vi "Control - Industrial Control.vi"() -> ()   [LabVIEW 2013, in "Control Workspace Object.lvlib"]
doc: "Sample numeric display item."
uses:
  Control Workspace Object.lvlib
  <vilib>/NI Veristand/Display Template Support/Display Template Support.llb/cluster_Screen Item Settings.ctl
  <vilib>/NI Veristand/Display Template Support/Display Template Support.llb/cluster_Graph Scale Settings.ctl
  <vilib>/NI Veristand/Display Template Support/Display Template Support.llb/cluster_Graph Plot Settings.ctl
  NationalInstruments.VeriStand.SystemStorage
  <vilib>/NI Veristand/Display Template Support/Display Template Support.llb/enum_Display Template Handler Minimal To Widget Msg.ctl
  <vilib>/NI Veristand/Display Template Support/Display Template Support.llb/enum_Display Template Handler Minimal To Workspace.ctl
  Shared/Types/Workspace Object State Variables.ctl
  Types/UI.Refs.ctl
  Shared/Types/UDP Streaming Command Cluster.ctl
  Shared/Types/UDP Streaming State.ctl
  Shared/Types/Workspace Object Cached Settings.ctl
  <vilib>/NI Veristand/Execution/Workspace/WorkspaceAPI.ctl
  <vilib>/NI Veristand/Execution/Workspace/SystemStateRegEventRef.ctl
  <vilib>/NI Veristand/Execution/Workspace/SystemStateEventRef.ctl
  <vilib>/NI Veristand/Display Template Support/Display Template Support.llb/sub_Display Template Handler Custom.vi
  Shared/Constants.vi
  <vilib>/NI Veristand/Execution/Workspace/NI VeriStand - Get Multiple Channel Values.vi
  <vilib>/NI Veristand/Execution/Workspace/NI VeriStand - Set Single Channel Value.vi
  Shared/Control Addon Shared.lvlib
  <vilib>/NI Veristand/Execution/Workspace/NI_VS Workspace ExecutionAPI.lvlib
  NationalInstruments.VeriStand.ClientAPI
panel:
  in  "Manual Value":bool
  in  "Revert":bool
  in  "Apply":bool
  in  "Manual Output":dbl
  in  "Manual Control":bool
  in  "Setpoint":dbl
  in  "NIVS.System Definition Root":refnum<k24>
  in  "NIVS.Gateway IP Address":string
  in  "Hold":bool
  in  "Autoscale Y":bool=TRUE
  in  "Autoscale X":bool=TRUE
  out "Chart":waveform(dbl)[](graph)
  out "Control Name":string
  in  "Item.Data":T1
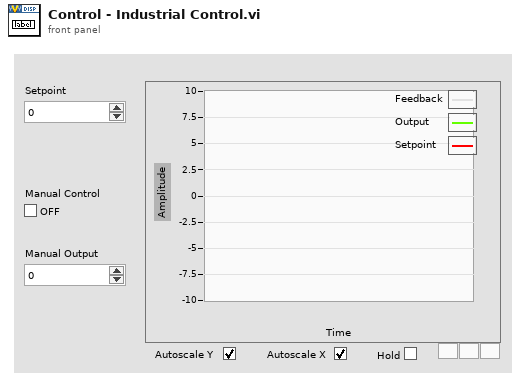
[diagram p1: front panel]
types:
  T1 = typedef "cluster_Screen Item Settings.ctl" = cluster{"Template VI":string, "Position X":i32, "Position Y":i32, "Custom":string, "Show Title Bar":bool, "ID":i32, "Always On Top":bool, "Allow Resize":bool, "Allow Minimize":bool, "Allow Close":bool, "Size to Screen":bool, "Screen.ID":i32, "State":enum16{"Normal", "New"}, "Title":string, "Window Bounds":cluster{"[0]":i16, "[1]":i16, "[2]":i16, "[3]":i16}, "Channel Ref":u64, "Unit":string, "Default Units?":bool, "Flash Limit?":bool, "Color 1":u32, "Color 2":u32, "Color 3":u32, "Color 4":u32, "Bck Color":u32, "Fore Color":u32, "Limit 1":dbl, "Limit 2":dbl, "Limit 3":dbl, "Limit 4":dbl, "Limit Mode 1":i32, "Limit Mode 2":i32, "Limit Mode 3":i32, "Limit Mode 4":i32, "Scale Precision":i32, "Scale Min":dbl, "Scale Max":dbl, "Format":i32, "Precision":i32, "Background Type":i32, "IDs":i32[], "Units":string[], "Labels":string[], "Scale Factor":dbl, "Scale Offset":dbl, "YScale Index":u32[], "XScale":T2, "YScales":T2[], "Plots":T3[], "Update Period":dbl, "History Length":dbl, "My.Ref":refnum<vi>, "Is Control?":bool, "Channel Paths":string[], "Custom Data":variant}
  T2 = typedef "cluster_Graph Scale Settings.ctl" = cluster{"Format":u8, "Precision":u8, "Fit":u8, "Label":string, "Use Default Label":bool, "Label Visible":bool, "Min":dbl, "Max":dbl}
  T3 = typedef "cluster_Graph Plot Settings.ctl" = cluster{"Bar Style":u8, "Fill To":i16, "Fill/PtColor":u32, "Line Style":u8, "Line Width":u8, "Color":u32, "Interp":u8, "Point Style":u8}
  T4 = typedef "Control Addon Shared.lvlib/Workspace Object State Variables.ctl" = cluster{"UI.Refs":T5, "Addon.GUID":string, "Addon.Name":string, "Addon.Type":enum16{"PID", "Industrial"}, "Data.UDPEngineQueue":refnum<queue>, "Data.Found?":bool, "Data.UDPChannels":string[], "Data.PreviousValues":dbl[], "Data.SlowChannels":string[], "Data.PendingChange?":bool, "CachedData.UserEvent":refnum<user-event>, "CachedData.Data":T6, "Workspace.Connected?":bool, "NIVS.SysDef":refnum<k24>, "NIVS.WorkspaceManager":T7, "NIVS.UserEventRefs":cluster{"Event Registration Refnum":refnum<event-registration>, "SystemChangeEventRef":T8}, "NIVS.SystemStateRefs":T9, "NIVS.LaunchRef":refnum<user-event>, "Setpoint Range":cluster{"Min":dbl, "Max":dbl}, "Output Range":cluster{"Min":dbl, "Max":dbl}}
  T5 = typedef "Control Addon Shared.lvlib/UI.Refs.ctl" = cluster{"Chart":refnum<vi>, "Manual Value":refnum<vi>, "Manual Output":refnum<vi>, "Revert":refnum<vi>, "Apply":refnum<vi>}
  T6 = typedef "Control Addon Shared.lvlib/Workspace Object Cached Settings.ctl" = cluster{"Path":string}
  T7 = typedef "NI_VS Workspace ExecutionAPI.lvlib/WorkspaceAPI.ctl" = refnum<k24>
  T8 = typedef "NI_VS Workspace ExecutionAPI.lvlib/SystemStateRegEventRef.ctl" = refnum<event-registration>
  T9 = typedef "NI_VS Workspace ExecutionAPI.lvlib/SystemStateEventRef.ctl" = cluster{"CustDatRef":refnum<user-event>, "EvtRef":refnum<k27>}
  T10 = typedef "enum_Display Template Handler Minimal To Workspace.ctl" = cluster{"Operation":enum16{"SetCustomData", "DeleteItem"}, "Data":variant}
  T11 = typedef "enum_Display Template Handler Minimal To Widget Msg.ctl" = enum16{"Stop", "LaunchConfigDialog"}
  T12 = typedef "Control Addon Shared.lvlib/UDP Streaming Command Cluster.ctl" = cluster{"Action":T13, "Channels":string[]}
  T13 = typedef "Control Addon Shared.lvlib/UDP Streaming State.ctl" = enum8{"Idle", "Start Acq", "Run", "Stop Acq", "Exit"}
  T14 = cluster{"Event Registration Refnum":refnum<event-registration>, "SystemChangeEventRef":T8}
  T15 = typedef "NI_VS Workspace ExecutionAPI.lvlib/SystemState.ctl" = u8
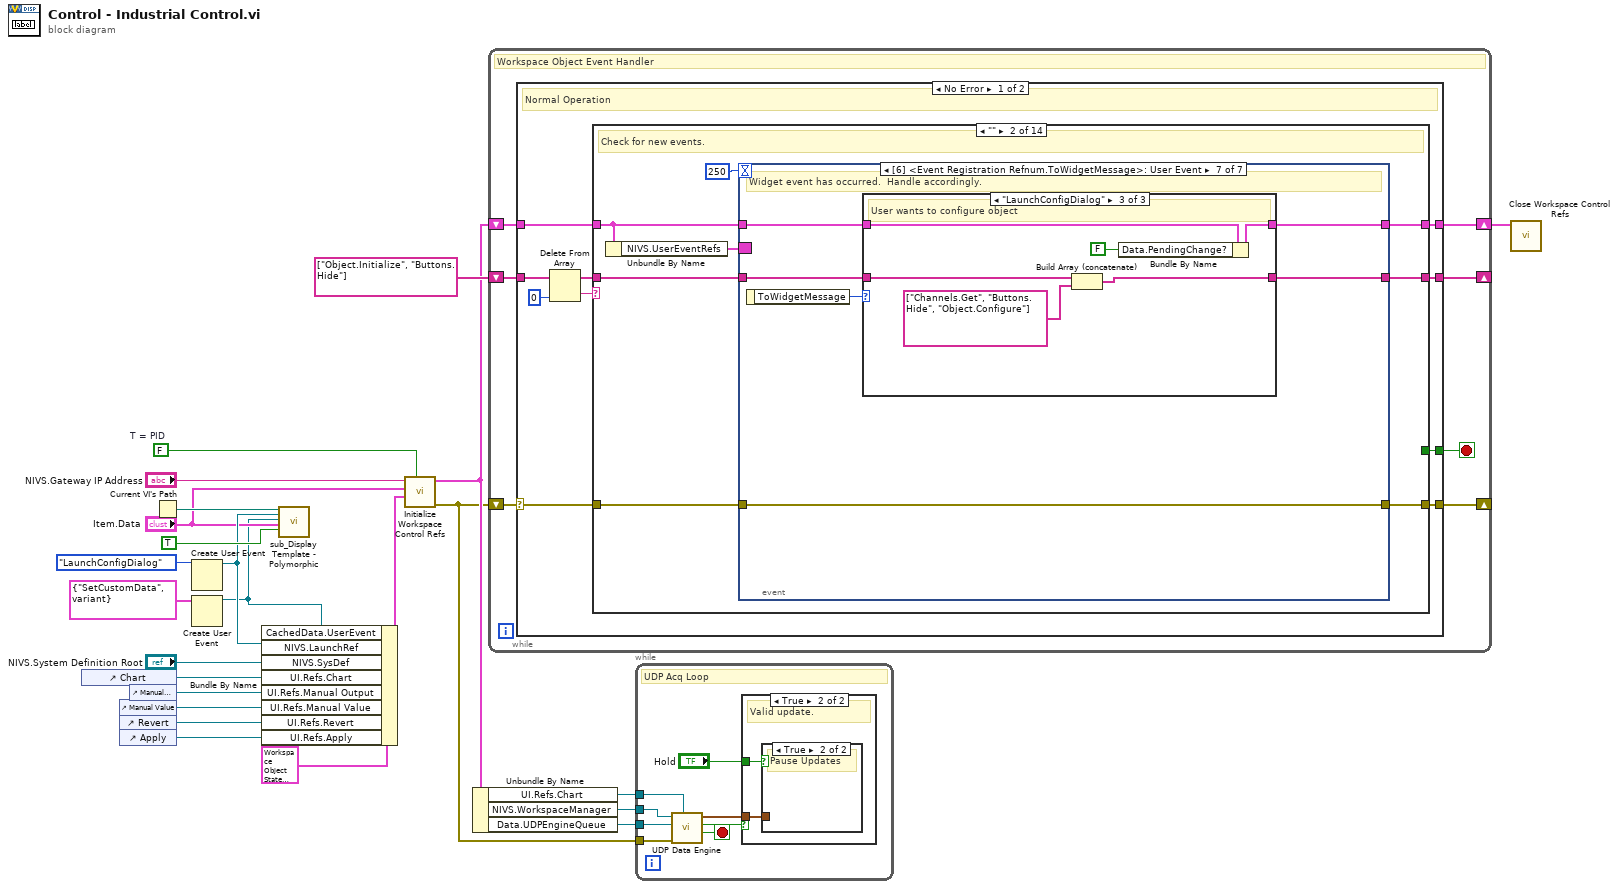
[diagram p0: block diagram]
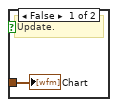
[diagram p3: hidden frame]
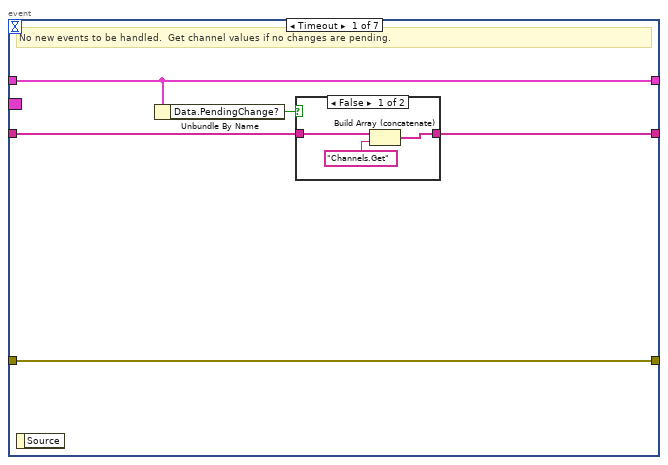
[diagram p5: hidden frame]
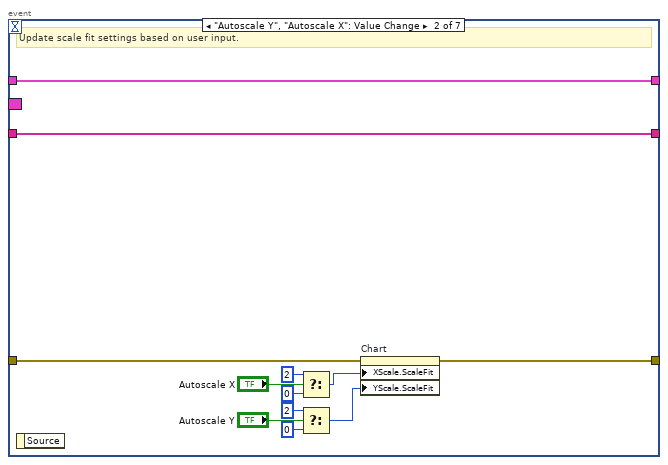
[diagram p7: hidden frame]
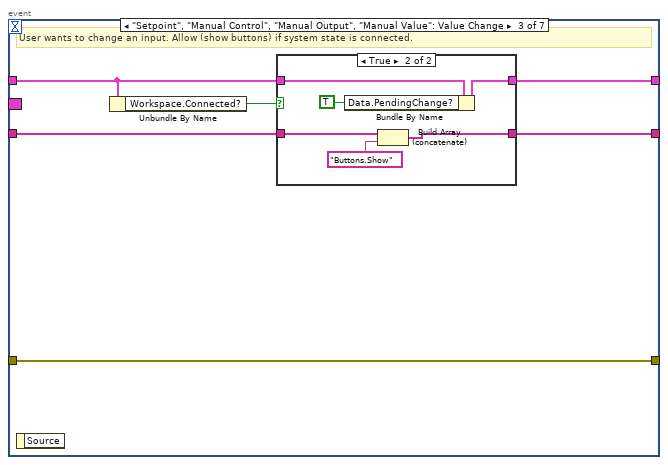
[diagram p8: hidden frame]
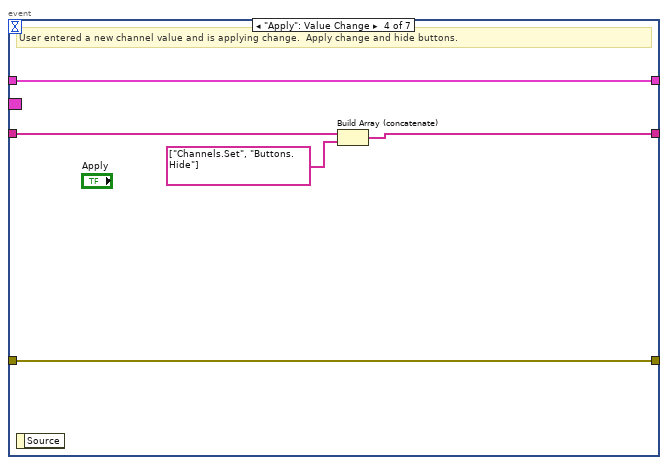
[diagram p10: hidden frame]
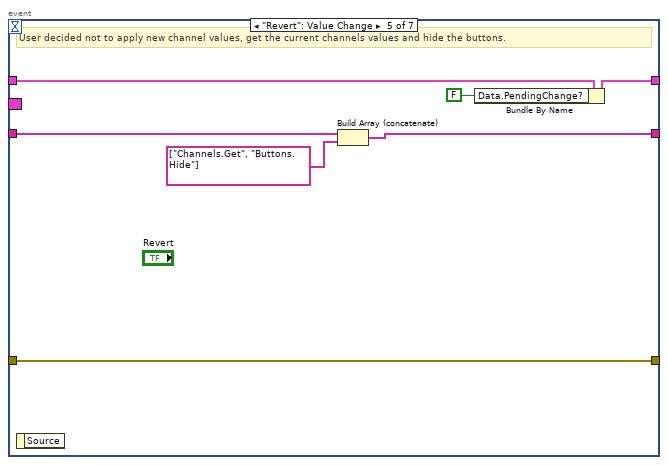
[diagram p11: hidden frame]
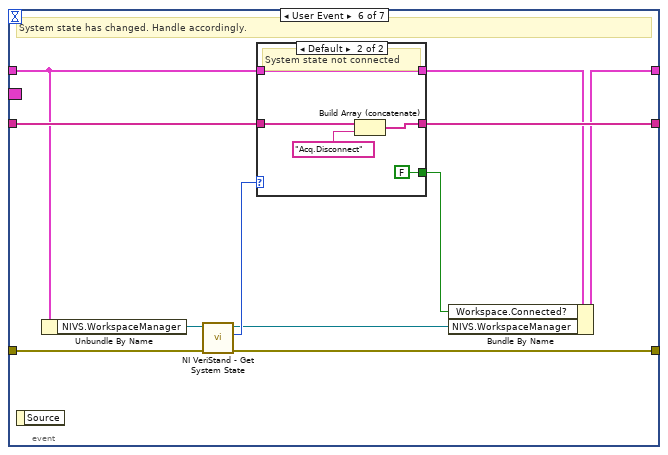
[diagram p12: hidden frame]
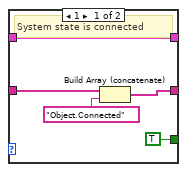
[diagram p13: hidden frame]
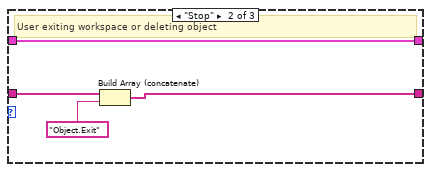
[diagram p15: hidden frame]
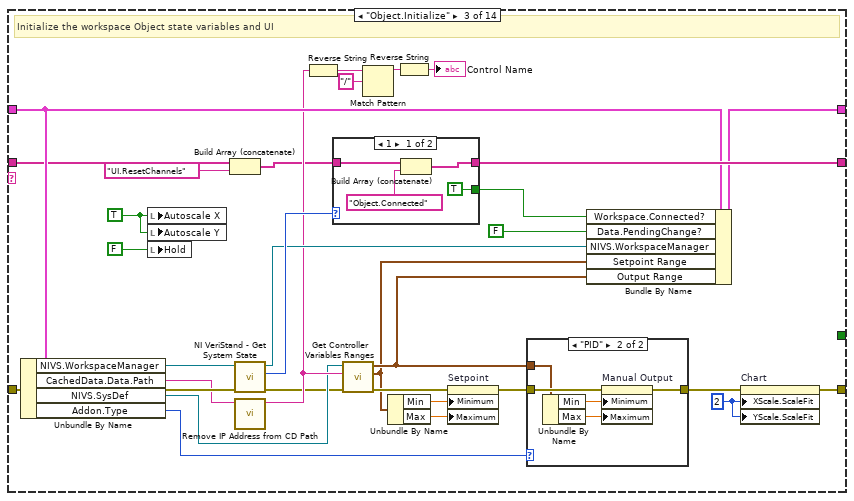
[diagram p16: hidden frame]
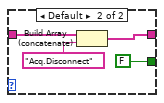
[diagram p18: hidden frame]
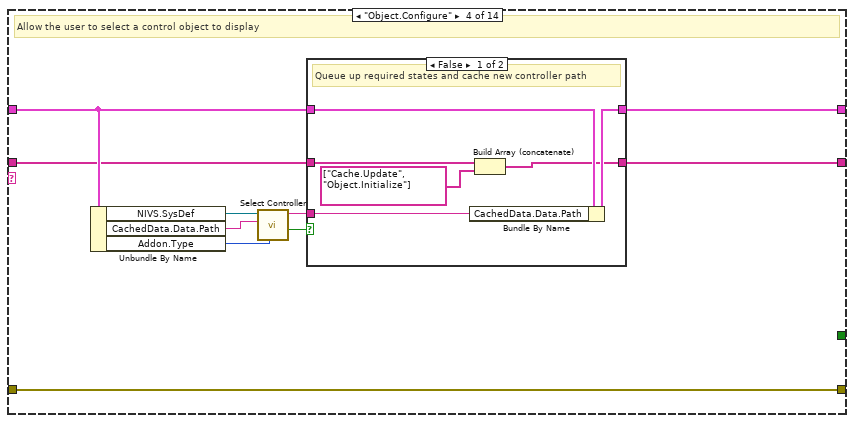
[diagram p19: hidden frame]
diagram:
  w6 = FALSE  # T = PID
  n1 = control-ref of="Chart"() -> (w12:refnum<vi>)
  n2 = control-ref of="Manual Value"() -> (w10:refnum<vi>)
  n3 = control-ref of="Revert"() -> (w9:refnum<vi>)
  n4 = control-ref of="Apply"() -> (w8:refnum<vi>)
  n5 = control-ref of="Manual Output"() -> (w11:refnum<vi>)
  n6 = Current VI's Path() -> (path=w22:path)
  n7 = Create User Event(user event datatype=enum_Display_Template_Handler_Minimal_To_Widget_Msg."LaunchConfigDialog" ("ToWidgetMessage")) -> (user event=w7:refnum<user-event>)  [unwired: 1 in, 1 out]
  n8 = Create User Event(user event datatype=T10 {"Operation"=enum."SetCustomData", "Data"=variant} ("Data")) -> (user event=w2:refnum<user-event>)  [unwired: 1 in, 1 out]
  n9 = Bundle By Name(cluster=T4 {"UI.Refs"={"Chart"=refnum, "Manual Value"=refnum, "Manual Output"=refnum, "Revert"=refnum, "Apply"=refnum}, "Addon.GUID"="", "Addon.Name"="", "Addon.Type"=enum."PID", "Data.UDPEngineQueue"=refnum, "Data.Found?"=FALSE, "Data.UDPChannels"=[], "Data.PreviousValues"=[], "Data.SlowChannels"=[], "Data.PendingChange?"=FALSE, "CachedData.UserEvent"=refnum, "CachedData.Data"={"Path"=""}, "Workspace.Connected?"=FALSE, "NIVS.SysDef"=refnum, "NIVS.WorkspaceManager"=refnum, "NIVS.UserEventRefs"={"Event Registration Refnum"=refnum, "SystemChangeEventRef"=refnum}, "NIVS.SystemStateRefs"={"CustDatRef"=refnum, "EvtRef"=refnum}, "NIVS.LaunchRef"=refnum, "Setpoint Range"={"Min"=0.0, "Max"=0.0}, "Output Range"={"Min"=0.0, "Max"=0.0}}, "CachedData.UserEvent"=w2, "NIVS.LaunchRef"=w7, "NIVS.SysDef"="NIVS.System Definition Root", "UI.Refs.Chart"=w12, "UI.Refs.Manual Output"=w11, "UI.Refs.Manual Value"=w10, "UI.Refs.Revert"=w9, "UI.Refs.Apply"=w8) -> (w4:T4)
  n10 = call-poly <vilib>:"sub_Display Template - Polymorphic.vi"("Parent.Path"=w22, "ToWidgetEvent"=w7, "ToWorkspace"=w2, "Item.Data"="Item.Data", "Resizable"=TRUE) -> ()  [unwired: 1 in, 14 out]
  n11 = call "Initialize Workspace Control Refs.vi"("T = PID"=w6, "State Variables in"=w4, "Item.Data"="Item.Data", "NIVS.Gateway IP Address"="NIVS.Gateway IP Address") -> ("error out"=w1:errorcluster, "State Variables out"=w15:T4)  [unwired: 6 in]
  n12 = Unbundle By Name(w15) -> ("UI.Refs.Chart"=w17:refnum<vi>, "NIVS.WorkspaceManager"=w16:T7, "Data.UDPEngineQueue"=w14:refnum<queue>)
  n13 = while {
    shift-right: [w29] -> _
    shift-left: string[] ["Object.Initialize", "Buttons.Hide"] -> [w30]
    shift-right: [w27] -> w19
    shift-left: w15 -> [w26]
    shift-right: [w28] -> _
    shift-left: w1 -> [w25]
    stop <- w31 stop-if-true
    # "Workspace Object Event Handler"
    n14 = case shown="No Error" w25 {
      selector: w25 -> [w32 w387]
      tunnel: [w41 _] -> w31
      tunnel: w30 -> [w39 w395]
      tunnel: [w36 w395] -> w29
      tunnel: [w35 w392] -> w28
      tunnel: [w34 w394] -> w27
      tunnel: w26 -> [w33 w394]
      frame No Error {
        # "Normal Operation"
        n15 = Delete From Array(array=w39, index=0) -> (deleted portion=w38:string, array with subset deleted=w37:string[])  [unwired: 1 in]
        n16 = case shown="\"\"" w38 {
          tunnel: [_ _ _ _ _ TRUE _ _ _ _ _ _ _ _] -> w41
          tunnel: [w44 w51 w168 w188 w212 w237 w244 w252 w254 w266 w272 w287 w347 w385] -> w36
          tunnel: w32 -> [w43 w49 w169 w194 w204 w232 w243 w247 w259 w262 w268 w284 w335 w384]
          tunnel: w37 -> [w44 w50 w140 w187 w223 w237 w244 w252 w260 w266 w272 w287 w347 w385]
          tunnel: w33 -> [w42 w45 w157 w192 w221 w229 w240 w251 w256 w265 w271 w277 w333 w382]
          tunnel: [w43 w48 w152 w194 w222 w231 w243 w246 w258 w261 w267 w283 w334 w384] -> w35
          tunnel: [w42 w47 w163 w191 w220 w229 w240 w251 w256 w265 w271 w282 w332 w382] -> w34
          frame Default {
            # "Do nothing."
          }
          frame "" {
            # "Check for new events."
            n17 = Unbundle By Name(w45) -> ("NIVS.UserEventRefs"=w46:T14)
            n18 = event shown="[6] <Event Registration Refnum.ToWidgetMessage>: User Event" {
              selector: w46 -> [_ _ _ _ _ _ _]
              dyn-events: _ -> [_ _ _ _ _ _ _]
              timeout: 250 -> [_ _ _ _ _ _ _]
              tunnel: [w55 w73 w76 w88 w96 w106 w125] -> w51
              tunnel: w50 -> [w56 w73 w77 w89 w97 w107 w124]
              tunnel: w49 -> [w57 w67 w79 w92 w99 w110 w123]
              tunnel: [w57 w66 w79 w92 w99 w109 w123] -> w48
              tunnel: [w54 w72 w78 w91 w94 w105 w121] -> w47
              tunnel: w45 -> [w54 w72 w75 w91 w95 w102 w122]
              event Timeout {
                # "No new events to be handled.  Get channel values if no changes are pending."
                n19 = event-data() -> ()  [unwired: 2 out]
                n20 = Unbundle By Name(w54) -> ("Data.PendingChange?"=w53:bool)
                n21 = case shown="False" w53 {
                  tunnel: w56 -> [w59 w61]
                  tunnel: [w58 w61] -> w55
                  frame False {
                    n22 = Build Array (concatenate)(w59, "Channels.Get") -> (w58:string[])
                  }
                  frame True {
                  }
                }
              }
              event "Autoscale Y", "Autoscale X": Value Change {
                # "Update scale fit settings based on user input."
                n23 = event-data() -> ()  [unwired: 2 out]
                n24 = Select(t=u8 2, s="Autoscale X", f=u8 0 ("X Scale.Scale Fit")) -> (s? t:f=w69:u8)
                n25 = Select(t=u8 2, s="Autoscale Y", f=u8 0 ("X Scale.Scale Fit")) -> (s? t:f=w62:u8)
                n26 = property on="Chart" class="WFChart (strict)"(error in=w67, "XScale.ScaleFit"=w69, "YScale.ScaleFit"=w62) -> (error out=w66:errorcluster)  [unwired: 1 in, 1 out]
              }
              event "Setpoint", "Manual Control", "Manual Output", "Manual Value": Value Change {
                # "User wants to change an input. Allow (show buttons) if system state is connected."
                n27 = event-data() -> ()  [unwired: 2 out]
                n28 = Unbundle By Name(w75) -> ("Workspace.Connected?"=w74:bool)
                n29 = case shown="True" w74 {
                  tunnel: w75 -> [w80 w86]
                  tunnel: [w80 w85] -> w78
                  tunnel: w77 -> [w81 w84]
                  tunnel: [w81 w82] -> w76
                  frame False {
                  }
                  frame True {
                    n30 = Bundle By Name(cluster=w86, "Data.PendingChange?"=TRUE ("Pending Change?")) -> (w85:T4)
                    n31 = Build Array (concatenate)(w84, "Buttons.Show") -> (w82:string[])
                  }
                }
              }
              event "Apply": Value Change {
                # "User entered a new channel value and is applying change.  Apply change and hide buttons."
                n32 = event-data() -> ()  [unwired: 2 out]
                n33 = Build Array (concatenate)(w89, string[] ["Channels.Set", "Buttons.Hide"]) -> (w88:string[])
              }
              event "Revert": Value Change {
                # "User decided not to apply new channel values, get the current channels values and hide the buttons."
                n34 = event-data() -> ()  [unwired: 2 out]
                n35 = Build Array (concatenate)(w97, string[] ["Channels.Get", "Buttons.Hide"]) -> (w96:string[])
                n36 = Bundle By Name(cluster=w95, "Data.PendingChange?"=FALSE ("Pending Change?")) -> (w94:T4)
              }
              event User Event {
                # "System state has changed. Handle accordingly."
                n37 = event-data() -> ()  [unwired: 2 out]
                n38 = Unbundle By Name(w102) -> ("NIVS.WorkspaceManager"=w101:T7)
                n39 = call <vilib>:"NI VeriStand - Get System State.vi"("error in (no error)"=w110, "WorkspaceManager in"=w101) -> ("error out"=w109:errorcluster, "System State"=w108:T15, "WorkspaceManager  out"=w100:T7)  [unwired: 5 in, 2 out]
                n40 = case shown="Default" w108 {
                  tunnel: w107 -> [w115 w120]
                  tunnel: [w114 w119] -> w106
                  tunnel: [w112 w117] -> w104
                  tunnel: w102 -> [w112 w117]
                  tunnel: [TRUE FALSE] -> w103
                  frame 1 {
                    # "System state is connected"
                    n41 = Build Array (concatenate)(w115, "Object.Connected") -> (w114:string[])
                  }
                  frame Default {
                    # "System state not connected"
                    n42 = Build Array (concatenate)(w120, "Acq.Disconnect") -> (w119:string[])
                  }
                }
                n43 = Bundle By Name(cluster=w104, "Workspace.Connected?"=w103, "NIVS.WorkspaceManager"=w100) -> (w105:T4)
              }
              event User Event {
                # "Widget event has occurred.  Handle accordingly."
                n44 = event-data() -> ("ToWidgetMessage"=w126:T11)  [unwired: 1 out]
                n45 = case shown="\"LaunchConfigDialog\"" w126 {
                  tunnel: [w128 w131 w137] -> w125
                  tunnel: w124 -> [w128 w132 w138]
                  tunnel: w122 -> [w127 w129 w134]
                  tunnel: [w127 w129 w133] -> w121
                  frame Default {
                    # "Do nothing."
                  }
                  frame "Stop" {
                    # "User exiting workspace or deleting object"
                    n46 = Build Array (concatenate)(w132, "Object.Exit") -> (w131:string[])
                  }
                  frame "LaunchConfigDialog" {
                    # "User wants to configure object"
                    n47 = Build Array (concatenate)(w138, string[] ["Channels.Get", "Buttons.Hide", "Object.Configure"]) -> (w137:string[])
                    n48 = Bundle By Name(cluster=w134, "Data.PendingChange?"=FALSE ("Pending Change?")) -> (w133:T4)
                  }
                }
              }
            }
          }
          frame "Object.Initialize" {
            w160 = u8 2 ("X Scale.Scale Fit")
            w161 = TRUE ("Autoscale X")
            # "Initialize the workspace Object state variables and UI"
            n49 = Unbundle By Name(w157) -> ("NIVS.WorkspaceManager"=w156:T7, "CachedData.Data.Path"=w150:string, "NIVS.SysDef"=w153:refnum<k24>, "Addon.Type"=w144:enum16{"PID", "Industrial"})
            n50 = local write "Autoscale X"(w161) -> ()
            n51 = local write "Autoscale Y"(w161) -> ()
            n52 = local write "Hold"(FALSE ("Hold")) -> ()
            n53 = Build Array (concatenate)(w140, "UI.ResetChannels") -> (w139:string[])
            n54 = call <vilib>:"NI VeriStand - Get System State.vi"("error in (no error)"=w169, "WorkspaceManager in"=w156) -> ("error out"=w151:errorcluster, "System State"=w170:T15, "WorkspaceManager  out"=w155:T7)  [unwired: 5 in, 2 out]
            n55 = call "Remove IP Address from CD Path.vi"("CD Path"=w150) -> ("Path"=w154:string)  [unwired: 10 in]
            n56 = Reverse String(1:w154) -> (0:w167:string)
            n57 = case shown="1" w170 {
              tunnel: w139 -> [w180 w184]
              tunnel: [w179 w183] -> w168
              tunnel: [TRUE FALSE] -> w162
              frame 1 {
                n58 = Build Array (concatenate)(w180, "Object.Connected") -> (w179:string[])
              }
              frame Default {
                n59 = Build Array (concatenate)(w184, "Acq.Disconnect") -> (w183:string[])
              }
            }
            n60 = call "Get Controller Variables Ranges.vi"("error in (no error)"=w151, "Path"=w154, "NIVS.SysDef Ref"=w153) -> ("error out"=w149:errorcluster, "Setpoint Range"=w142:cluster{"Min":dbl, "Max":dbl}, "Output Range"=w143:cluster{"Min":dbl, "Max":dbl})  [unwired: 6 in]
            n61 = Match Pattern(string=w167, regular expression="/") -> (before substring=w164:string)  [unwired: 1 in, 3 out]
            n62 = Unbundle By Name(w142) -> ("Min"=w148:dbl, "Max"=w147:dbl)
            n63 = Reverse String(1:w164) -> (0:→"Control Name":string)
            n64 = property on="Setpoint" class="DigNum (strict)"(error in=w149, "Minimum"=w148, "Maximum"=w147) -> (error out=w146:errorcluster)  [unwired: 1 in, 1 out]
            n65 = case shown="\"PID\"" w144 {
              tunnel: w146 -> [w171 w176]
              tunnel: [w171 w175] -> w145
              tunnel: w143 -> [_ w174]
              frame Default {
              }
              frame "PID" {
                n66 = Unbundle By Name(w174) -> ("Min"=w173:dbl, "Max"=w172:dbl)
                n67 = property on="Manual Output" class="DigNum (strict)"(error in=w176, "Minimum"=w173, "Maximum"=w172) -> (error out=w175:errorcluster)  [unwired: 1 in, 1 out]
              }
            }
            n68 = Bundle By Name(cluster=w157, "Workspace.Connected?"=w162, "Data.PendingChange?"=FALSE ("Pending Change?"), "NIVS.WorkspaceManager"=w155, "Setpoint Range"=w142, "Output Range"=w143) -> (w163:T4)
            n69 = property on="Chart" class="WFChart (strict)"(error in=w145, "XScale.ScaleFit"=w160, "YScale.ScaleFit"=w160) -> (error out=w152:errorcluster)  [unwired: 1 in, 1 out]
          }
          frame "Object.Configure" {
            # "Allow the user to select a control object to display"
            n70 = Unbundle By Name(w192) -> ("NIVS.SysDef"=w186:refnum<k24>, "CachedData.Data.Path"=w193:string, "Addon.Type"=w185:enum16{"PID", "Industrial"})
            n71 = call "Select Controller.vi"("Type"=w185, "CD Path"=w193, "NIVS.System Definition Root"=w186) -> ("Cancelled?"=w190:bool, "Custom Device Path Out"=w189:string)  [unwired: 6 in, 1 out]
            n72 = case shown="False" w190 {
              tunnel: w192 -> [w200 w201]
              tunnel: [w199 w201] -> w191
              tunnel: w189 -> [w198 _]
              tunnel: [w196 w202] -> w188
              tunnel: w187 -> [w197 w202]
              frame False {
                # "Queue up required states and cache new controller path"
                n73 = Bundle By Name(cluster=w200, "CachedData.Data.Path"=w198) -> (w199:T4)
                n74 = Build Array (concatenate)(w197, string[] ["Cache.Update", "Object.Initialize"]) -> (w196:string[])
              }
              frame True {
                # "User canceled"
              }
            }
          }
          frame "Object.Connected" {
            w209 = "/" ("string")
            # "System state is Connected. Get path to required channels and start UDP acquisition if channels found."
            n75 = Unbundle By Name(w221) -> ("NIVS.SysDef"=w205:refnum<k24>, "CachedData.Data.Path"=w219:string, "Addon.Name"=w206:string, "Addon.GUID"=w203:string)
            n76 = global read "Constants.vi" "Name.ManualControl"() -> (w218:string)
            n77 = global read "Constants.vi" "Name.Channels"() -> (w208:string)
            n78 = call "Remove IP Address from CD Path.vi"("CD Path"=w219) -> ("Path"=w217:string)  [unwired: 10 in]
            n79 = Concatenate Strings(w217, w209, w208, w209, w218) -> (w216:string)
            n80 = Concatenate Strings(w217, w209, w208, w209, w206) -> (w215:string)
            n81 = call "Get Dependent Nodes from SysDef Root.vi"("error in (no error)"=w204, "GUID"=w203, "Path"=w217, "SysDef Ref"=w205) -> ("error out"=w222:errorcluster, "Channels"=w211:string[], "Found"=w207:bool)  [unwired: 5 in]
            n82 = case shown="True" w207 {
              tunnel: w223 -> [w224 w227]
              tunnel: [w224 w226] -> w212
              frame False {
              }
              frame True {
                n83 = Build Array (concatenate)(w227, "Acq.Start") -> (w226:string[])
              }
            }
            n84 = Index Array(array=w211, index=2) -> (element=w213:string)
            n85 = Build Array(w213, w216, w215) -> (w210:string[])
            n86 = Bundle By Name(cluster=w221, "Data.Found?"=w207, "Data.UDPChannels"=w211, "Data.SlowChannels"=w210) -> (w220:T4)
          }
          frame "Object.Exit" {
            # "Stop current loop.  Queue Stop Acq and Exit to UDP loop."
            n87 = Unbundle By Name(w229) -> ("Data.UDPEngineQueue"=w228:refnum<queue>)
            n88 = Enqueue Element(queue=w228, element=T12 {"Action"=enum."Stop Acq", "Channels"=[]}, error in (no error)=w232) -> (queue out=w235:refnum<queue>, error out=w233:errorcluster)  [unwired: 1 in, 1 out]
            n89 = Enqueue Element(queue=w235, element=T12 {"Action"=enum."Exit", "Channels"=[]}, error in (no error)=w233) -> (error out=w231:errorcluster)  [unwired: 1 in, 2 out]
          }
          frame "Cache.Update" {
            # "Cache any data needing to be permenantly stored with the workspace object."
            n90 = Unbundle By Name(w240) -> ("CachedData.UserEvent"=w238:refnum<user-event>, "CachedData.Data"=w239:T6)
            n91 = Bundle By Name(cluster=T10 {"Operation"=enum."SetCustomData", "Data"=variant} ("event data"), "Data"=w239) -> (w241:T10)
            n92 = Generate User Event(user event=w238, event data cluster=w241) -> ()  [unwired: 2 in, 2 out]
          }
          frame "Acq.Start" {
            # "Send a Start Acq command to the UDP Loop.  Include the channels to  monitor."
            n93 = Unbundle By Name(w251) -> ("Data.UDPEngineQueue"=w245:refnum<queue>, "Data.UDPChannels"=w249:string[])
            n94 = Bundle By Name(cluster=T12 {"Action"=enum."Start Acq", "Channels"=[]}, "Channels"=w249) -> (w248:T12)
            n95 = Enqueue Element(queue=w245, element=w248, error in (no error)=w247) -> (error out=w246:errorcluster)  [unwired: 1 in, 2 out]
          }
          frame "Acq.Disconnect" {
            # "Send Stop Acq to the UDP Acq Loop.  Reset the UI."
            n96 = Unbundle By Name(w256) -> ("Data.UDPEngineQueue"=w255:refnum<queue>)
            n97 = Enqueue Element(queue=w255, element=T12 {"Action"=enum."Stop Acq", "Channels"=[]}, error in (no error)=w259) -> (error out=w258:errorcluster)  [unwired: 1 in, 2 out]
            n98 = Build Array (concatenate)(w260, "UI.ResetChannels") -> (w254:string[])
          }
          frame "Buttons.Hide" {
            w263 = FALSE ("Hold")
            # "Hide the apply and revert buttons from the user."
            n99 = property on="Apply" class="Bool"(error in=w262, "Visible"=w263) -> (error out=w264:errorcluster)  [unwired: 1 in, 1 out]
            n100 = property on="Revert" class="Bool"(error in=w264, "Visible"=w263) -> (error out=w261:errorcluster)  [unwired: 1 in, 1 out]
          }
          frame "Buttons.Show" {
            w269 = TRUE ("Hold")
            # "Show the apply and revert buttons to the user."
            n101 = property on="Apply" class="Bool"(error in=w268, "Visible"=w269) -> (error out=w270:errorcluster)  [unwired: 1 in, 1 out]
            n102 = property on="Revert" class="Bool"(error in=w270, "Visible"=w269) -> (error out=w267:errorcluster)  [unwired: 1 in, 1 out]
          }
          frame "Channels.Get" {
            # "Get the current slow speed channel values from VeriStand if no pending change, data paths are valid and system state is connected."
            n103 = Unbundle By Name(w277) -> ("Setpoint Range.Max"=w276:dbl, "Setpoint Range.Min"=w275:dbl, "Data.PendingChange?"=w278:bool, "Output Range.Max"=w274:dbl, "Output Range.Min"=w273:dbl, "Addon.Type"=w281:enum16{"PID", "Industrial"}, "Data.Found?"=w285:bool, "Workspace.Connected?"=w286:bool, "NIVS.WorkspaceManager"=w280:T7, "Data.SlowChannels"=w279:string[])
            n104 = case shown="False" w278 {
              tunnel: w286 -> [w309 _]
              tunnel: w285 -> [w303 _]
              tunnel: w284 -> [w300 w326]
              tunnel: [w299 w326] -> w283
              tunnel: [w298 w327] -> w282
              tunnel: w281 -> [w297 _]
              tunnel: w280 -> [w296 _]
              tunnel: w279 -> [w294 _]
              tunnel: w277 -> [w293 w327]
              tunnel: w276 -> [w291 _]
              tunnel: w275 -> [w290 _]
              tunnel: w274 -> [w289 _]
              tunnel: w273 -> [w288 _]
              frame False {
                # "No pending data change.  Allow for a get."
                n105 = Compound Arithmetic op=AND(w303, w309) -> (w304:bool)
                n106 = case shown="True" w304 {
                  tunnel: w300 -> [w319 w325]
                  tunnel: [w319 w324] -> w299
                  tunnel: w296 -> [w318 w323]
                  tunnel: [w318 w322] -> w295
                  tunnel: w294 -> [_ w321]
                  tunnel: [dbl[] [0.0, 0.0, 0.0] ("Values") w320] -> w308
                  frame False {
                    # "Do Nothing."
                  }
                  frame True {
                    # "Connected & paths valid"
                    n107 = call-poly <vilib>:"NI VeriStand - Get Channel Value.vi"("error in (no error)"=w325, "Channels"=w321, "WorkspaceManager in"=w323) -> ("error out"=w324:errorcluster, "Values"=w320:dbl[], "WorkspaceManager out"=w322:T7)  [unwired: 6 in]
                  }
                }
                n108 = Index Array(array=w308) -> (element #1=w307:dbl, element #2=w302:dbl, element #3=w301:dbl)  [unwired: 3 in]
                n109 = case shown="\"PID\"" w297 {
                  tunnel: w301 -> [w311 w316]
                  tunnel: w289 -> [_ w314]
                  tunnel: w288 -> [_ w313]
                  frame "Industrial" {
                    n110 = To Long Integer(number=w311) -> (32bit integer=w312:i32)
                    n111 = Not Equal To 0?(x=w312) -> (x != 0?=w310:bool)
                    n112 = local write "Manual Value"(w310) -> ()
                  }
                  frame "PID" {
                    n113 = In Range and Coerce(upper limit=w314, x=w316, lower limit=w313) -> (coerced(x)=w315:dbl)  [unwired: 1 out]
                    n114 = local write "Manual Output"(w315) -> ()
                  }
                }
                n115 = To Long Integer(number=w302) -> (32bit integer=w306:i32)
                n116 = In Range and Coerce(upper limit=w291, x=w307, lower limit=w290) -> (coerced(x)=w292:dbl)  [unwired: 1 out]
                n117 = Not Equal To 0?(x=w306) -> (x != 0?=w305:bool)
                n118 = local write "Setpoint"(w292) -> ()
                n119 = local write "Manual Control"(w305) -> ()
                n120 = Bundle By Name(cluster=w293, "NIVS.WorkspaceManager"=w295, "Data.PreviousValues"=w308) -> (w298:T4)
              }
              frame True {
                # "A change is pending.  Don't get channels as this would overwrite the pending change."
              }
            }
          }
          frame "Channels.Set" {
            # "Set Channels if data paths are valid and system state is connected and there is a change in the data value."
            n121 = Unbundle By Name(w333) -> ("Data.Found?"=w338:bool, "Workspace.Connected?"=w341:bool, "Data.PreviousValues"=w340:dbl[], "Data.SlowChannels"=w342:string[], "NIVS.WorkspaceManager"=w330:T7, "Addon.Type"=w328:enum16{"PID", "Industrial"})
            n122 = case shown="\"PID\"" w328 {
              tunnel: [w349 "Manual Output"] -> w336
              frame "Industrial" {
                n123 = Boolean To (0,1)(Boolean="Manual Value") -> (0, 1=w349:i16)
              }
              frame "PID" {
              }
            }
            n124 = Boolean To (0,1)(Boolean="Manual Control") -> (0, 1=w337:i16)
            n125 = Build Array("Setpoint", w337, w336) -> (w343:dbl[])
            n126 = Not Equal?(x=w340, y=w343) -> (x != y?=w346:bool[])
            n127 = Compound Arithmetic op=AND(w338, w341) -> (w339:bool)
            n128 = case shown="True" w339 {
              tunnel: w346 -> [_ w359]
              tunnel: w343 -> [_ w358]
              tunnel: w335 -> [w352 w357]
              tunnel: [w352 w356] -> w334
              tunnel: w330 -> [w351 w355]
              tunnel: [w351 w354] -> w329
              tunnel: w342 -> [_ w353]
              frame False {
                # "Do nothing"
              }
              frame True {
                # "Connected & paths valid"
                n129 = for {
                  shift-right: [w365] -> w356
                  shift-left: w357 -> [w366]
                  shift-right: [w364] -> w354
                  shift-left: w355 -> [w363]
                  tunnel: w359 -> [w362] mode=indexing
                  tunnel: w358 -> [w361] mode=indexing
                  tunnel: w353 -> [w360] mode=indexing
                  n130 = case shown="False" w362 {
                    tunnel: w366 -> [w368 w374]
                    tunnel: [w368 w373] -> w365
                    tunnel: [w367 w372] -> w364
                    tunnel: w363 -> [w367 w371]
                    tunnel: w361 -> [_ w370]
                    tunnel: w360 -> [_ w369]
                    frame False {
                      # "Do nothing"
                    }
                    frame True {
                      # "Update channel"
                      n131 = call-poly <vilib>:"NI VeriStand - Set Channel Value.vi"("error in (no error)"=w374, "Value"=w370, "Channel"=w369, "WorkspaceManager in"=w371) -> ("error out"=w373:errorcluster, "WorkspaceManager out"=w372:T7)  [unwired: 6 in]
                    }
                  }
                }
              }
            }
            n132 = Bundle By Name(cluster=w333, "Data.PendingChange?"=FALSE ("Pending Change?"), "NIVS.WorkspaceManager"=w329) -> (w332:T4)
          }
          frame "UI.ResetChannels" {
            w383 = FALSE ("Manual Control")
            w377 = 0.0 ("Setpoint")
            # "Reset slow speed channel displayed values."
            n133 = Unbundle By Name(w382) -> ("Setpoint Range.Max"=w381:dbl, "Setpoint Range.Min"=w380:dbl, "Output Range.Max"=w379:dbl, "Output Range.Min"=w378:dbl)
            n134 = In Range and Coerce(upper limit=w381, x=w377, lower limit=w380) -> (coerced(x)=w376:dbl)  [unwired: 1 out]
            n135 = In Range and Coerce(upper limit=w379, x=w377, lower limit=w378) -> (coerced(x)=w375:dbl)  [unwired: 1 out]
            n136 = local write "Setpoint"(w376) -> ()
            n137 = local write "Manual Output"(w375) -> ()
            n138 = local write "Manual Control"(w383) -> ()
            n139 = local write "Manual Value"(w383) -> ()
          }
        }
      }
      frame Error {
        # "Handle Errors."
        n140 = Unbundle By Name(w387) -> ("code"=w391:i32)
        n141 = Equal?(x=-307654, y=w391) -> (x = y?=w389:bool)
        n142 = Select(t=errorcluster {"status"=FALSE, "code"=0, "source"=""}, s=w389, f=w387) -> (s? t:f=w386:errorcluster)
        n143 = call <vilib>:"Simple Error Handler.vi"("error in (no error)"=w386) -> ("error out"=w393:errorcluster)  [unwired: 4 in, 4 out]
        n144 = call <vilib>:"Clear Errors.vi"("error in (no error)"=w393) -> ("error out"=w392:errorcluster)  [unwired: 6 in]
      }
    }
  }
  n145 = while {
    tunnel: w16 -> [w398]
    tunnel: w14 -> [w403]
    tunnel: w17 -> [w399]
    tunnel: w1 -> [w397]
    stop <- w402 stop-if-true
    # "UDP Acq Loop"
    n146 = call "UDP Data Engine.vi"("WaveformChart Ref"=w399, "error in (no error)"=w397, "UDP Engine Queue"=w403, "WorkspaceManager"=w398) -> ("Exit"=w402:bool, "Update?"=w396:bool, "Waveform"=w400:waveform(dbl)[])  [unwired: 4 in, 1 out]
    n147 = case shown="True" w396 {
      tunnel: "Hold" -> [_ w405]
      tunnel: w400 -> [_ w404]
      frame False {
        # "Do Nothing."
      }
      frame True {
        # "Valid update."
        n148 = case shown="True" w405 {
          tunnel: w404 -> [w406 _]
          frame False {
            # "Update."
            "Chart" <- w406
          }
          frame True {
            # "Pause Updates"
          }
        }
      }
    }
  }
  n149 = call "Close Workspace Control Refs.vi"("State Variables in"=w19) -> ()  [unwired: 11 in]
